vi "PipBoy_SetImage.vi"(7 "Function":string, 8 "error in (no error)":errorcluster, 9 "Image to draw":i32, 10 "Icon":u16[][](array[numeric]), 11 "VisaPic32In":refnum<visa-resource-name>) -> (0 "error out":errorcluster, 3 "VisaPic32Out":refnum<visa-resource-name>)   [LabVIEW 2014]
uses:
  <vilib>/Utility/error.llb/Error Cluster From Error Code.vi
  <vilib>/ErrorRing/Error Ring.xnode
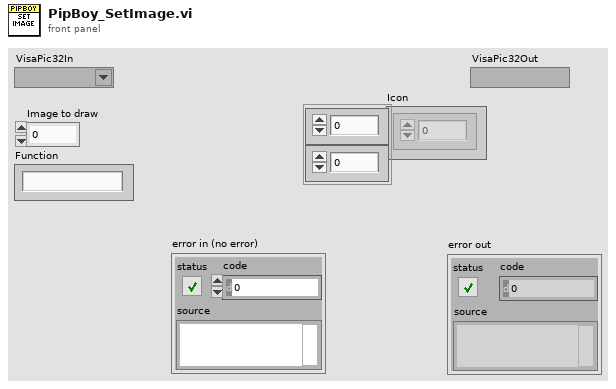
[diagram p1: front panel]
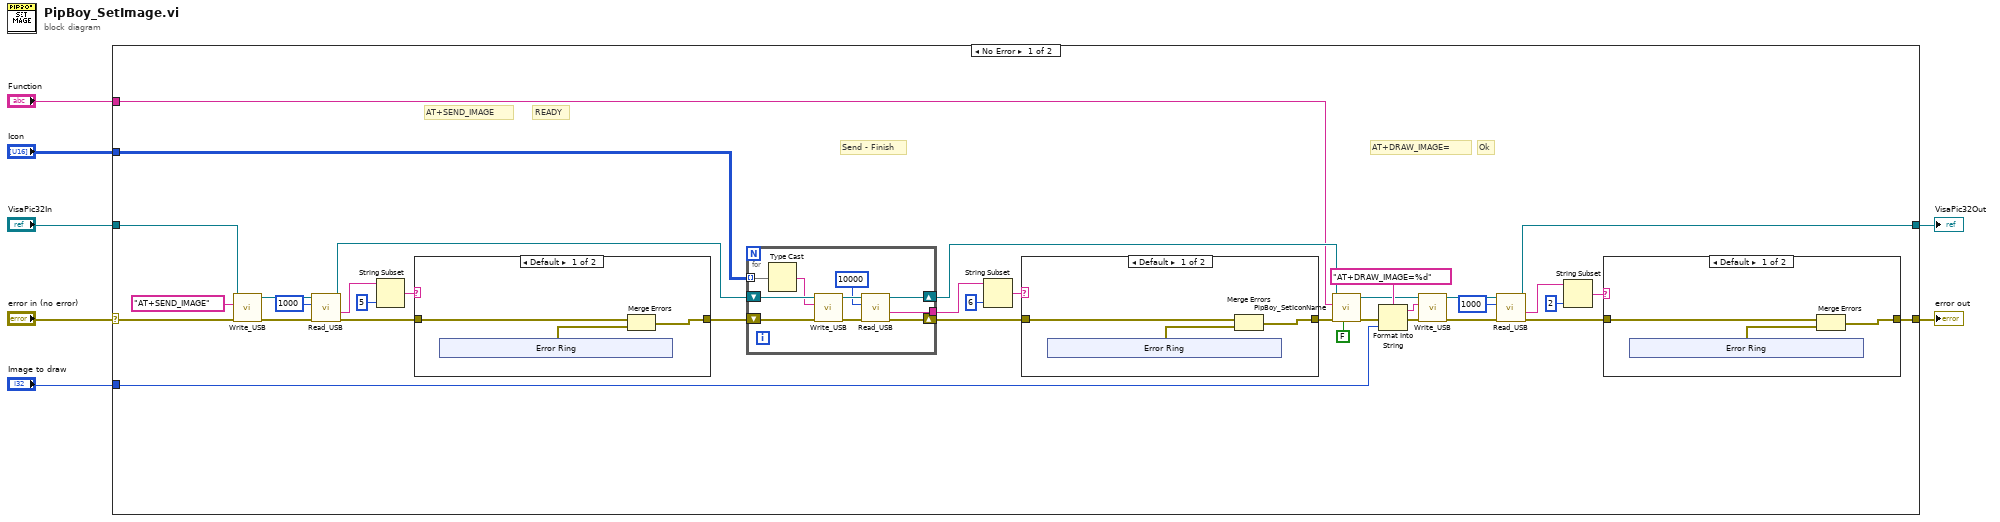
[diagram p0: block diagram]
diagram:
  n1 = case shown="No Error" "error in (no error)" {
    selector: "error in (no error)" -> [w36 w82]
    tunnel: [w27 w82] -> w6
    tunnel: [w32 w81] -> w5
    tunnel: "Icon" -> [w31 _]
    tunnel: "VisaPic32In" -> [w30 w81]
    tunnel: "Image to draw" -> [w29 _]
    tunnel: "Function" -> [w8 _]
    frame No Error {
      # "READY"
      # "Send - Finish"
      # "AT+SEND_IMAGE"
      # "Ok"
      # "AT+DRAW_IMAGE="
      n2 = call "Write_USB.vi"("entrée d'erreur"=w36, "buffer d'écriture"="AT+SEND_IMAGE", "Nom de ressource VISA"=w30) -> ("sortie d'erreur"=w38:errorcluster, "Nom de ressource VISA en sortie"=w39:refnum<visa-resource-name>)  [unwired: 7 in]
      n3 = call "Read_USB.vi"("entrée d'erreur"=w38, "timeout (0)"=u32 1000, "Nom de ressource VISA"=w39) -> ("sortie d'erreur"=w26:errorcluster, "chaîne en sortie"=w20:string, "Nom de ressource VISA en sortie"=w15:refnum<visa-resource-name>)  [unwired: 6 in]
      n4 = String Subset(string=w20, length (rest)=5 ("length (rest)")) -> (substring=w19:string)  [unwired: 1 in]
      n5 = case shown="Default" w19 {
        tunnel: [w54 w61] -> w24
        tunnel: w26 -> [w55 w61]
        frame Default {
          n6 = xnode "Error Ring"() -> ("error out"=w53:errorcluster)
          n7 = Merge Errors(w55, w53) -> (w54:errorcluster)
        }
        frame "READY" {
        }
      }
      n8 = for {
        tunnel: w31 -> [w79] mode=indexing
        shift-right: [w74] -> w25
        shift-left: w24 -> [w78]
        shift-right: [w76] -> w11
        shift-left: w15 -> [w80]
        tunnel: [w71] -> w23
        n9 = Type Cast(x=w79) -> (*(type *) &x=w72:string)  [unwired: 1 in]
        n10 = call "Write_USB.vi"("entrée d'erreur"=w78, "buffer d'écriture"=w72, "Nom de ressource VISA"=w80) -> ("sortie d'erreur"=w75:errorcluster, "Nom de ressource VISA en sortie"=w77:refnum<visa-resource-name>)  [unwired: 7 in]
        n11 = call "Read_USB.vi"("entrée d'erreur"=w75, "timeout (0)"=u32 10000, "Nom de ressource VISA"=w77) -> ("sortie d'erreur"=w74:errorcluster, "chaîne en sortie"=w71:string, "Nom de ressource VISA en sortie"=w76:refnum<visa-resource-name>)  [unwired: 6 in]
      }
      n12 = String Subset(string=w23, length (rest)=6 ("length (rest)")) -> (substring=w14:string)  [unwired: 1 in]
      n13 = case shown="Default" w14 {
        tunnel: [w45 w52] -> w13
        tunnel: w25 -> [w46 w52]
        frame Default {
          n14 = xnode "Error Ring"() -> ("error out"=w44:errorcluster)
          n15 = Merge Errors(w46, w44) -> (w45:errorcluster)
        }
        frame "FINISH" {
        }
      }
      n16 = call "PipBoy_SetIconName.vi"("DrawIcon?"=FALSE, "error in (no error)"=w13, "Function"=w8, "VisaPic32In"=w11) -> ("error out"=w12:errorcluster, "VisaPic32Out"=w10:refnum<visa-resource-name>)  [unwired: 6 in]
      n17 = Format Into String(format string="AT+DRAW_IMAGE=%d", error in=w12, w29) -> (resulting string=w40:string, error out=w42:errorcluster)  [unwired: 1 in]
      n18 = call "Write_USB.vi"("entrée d'erreur"=w42, "buffer d'écriture"=w40, "Nom de ressource VISA"=w10) -> ("sortie d'erreur"=w33:errorcluster, "Nom de ressource VISA en sortie"=w35:refnum<visa-resource-name>)  [unwired: 7 in]
      n19 = call "Read_USB.vi"("entrée d'erreur"=w33, "timeout (0)"=u32 1000, "Nom de ressource VISA"=w35) -> ("sortie d'erreur"=w28:errorcluster, "chaîne en sortie"=w17:string, "Nom de ressource VISA en sortie"=w32:refnum<visa-resource-name>)  [unwired: 6 in]
      n20 = String Subset(string=w17, length (rest)=2 ("length (rest)")) -> (substring=w16:string)  [unwired: 1 in]
      n21 = case shown="Default" w16 {
        tunnel: [w63 w70] -> w27
        tunnel: w28 -> [w64 w70]
        frame Default {
          n22 = xnode "Error Ring"() -> ("error out"=w62:errorcluster)
          n23 = Merge Errors(w64, w62) -> (w63:errorcluster)
        }
        frame "OK" {
        }
      }
    }
    frame Error {
    }
  }
  "error out" <- w6
  "VisaPic32Out" <- w5
